vi "Chart (SubVI).vi"(10 "data":string, 11 "Sign bytes":string) -> (2 "Numeric":i32, 3 "Chart":i32(graph))   [LabVIEW 2012]
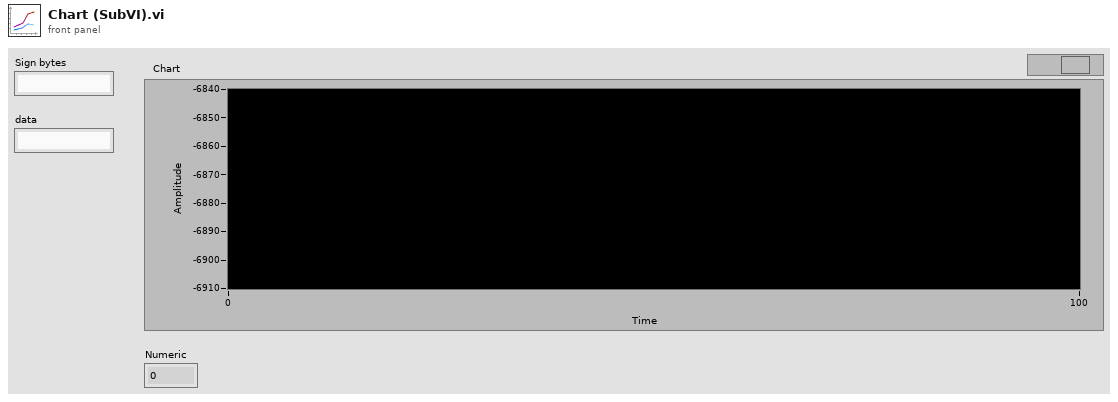
[diagram p1: front panel]
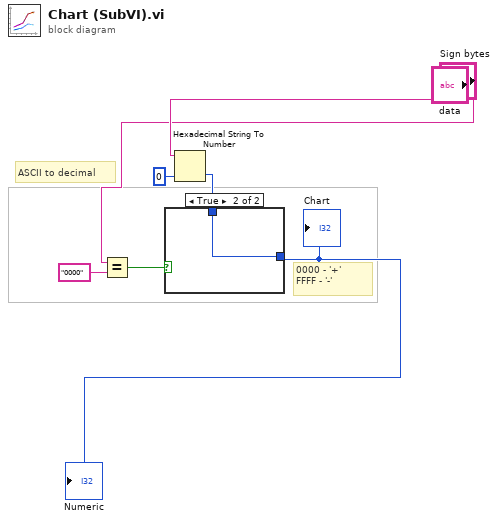
[diagram p0: block diagram]
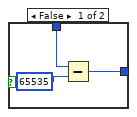
[diagram p2: hidden frame]
diagram:
  # "0000 - '+'\nFFFF - '-'"
  # "ASCII to decimal"
  n1 = Equal?(x="Sign bytes", y="0000") -> (x = y?=w5:bool)
  n2 = Hexadecimal String To Number(string="data", default (0uL)=0 ("default (0 U32)")) -> (number=w2:i32)  [unwired: 1 in, 1 out]
  n3 = case shown="True" w5 {
    tunnel: w2 -> [w9 w11]
    tunnel: [w10 w11] -> w7
    frame False {
      n4 = Subtract(x=w9, y=65535) -> (x-y=w10:i32)
    }
    frame True {
    }
  }
  "Chart" <- w7
  "Numeric" <- w7
